vi "dischargetest.vi"(8 "error in":errorcluster, 9 "Serial Configuration":T1={"Baud Rate"=9600, "Parity"=0, "Data Bits"=8, "Stop Bits"=10, "Flow Control"=0} {"Flow Control" items=["None", "XON/XOFF", "RTS/CTS", "XON/XOFF & RTS/CTS", "DTR/DSR", "XON/XOFF & DTR/DSR"]; "Stop Bits" items=["1.0"=10, "1.5"=15, "2.0"=20]; "Data Bits" items=["7"=7, "8"=8]; "Parity" items=["None", "Odd", "Even", "Mark", "Space"]; "Baud Rate" items=["300"=300, "600"=600, "1200"=1200, "2400"=2400, "4800"=4800, "9600"=9600, "19200"=19200]}, 11 "VISA resource name":refnum<visa-resource-name>) -> ()   [LabVIEW 2020]
uses:
  <instrlib>/IT-M3400/IT-M3400.lvlib
panel:
  out "Read Current(A)":dbl format="%.2g"
  out "Read Voltage(V)":dbl format="%.2g"
  in  "stop":bool
  in  "Save File(1-10)":u8=1 min=1 max=10 step=1
  in  "Stop Time(s)":dbl
  in  "Stop Capacity(Ah)":dbl
  in  "Stop Current(A)":dbl
  in  "Stop Voltage(V)":dbl
  in  "Battery Mode":u8(ring) items=["Charge", "Discharge"]
  in  "Discharge Current(A)":dbl
  in  "Discharge Voltage(V)":dbl
  in  "Channel":i32(ring)=1 items=["Channel 1"=1, "Channel 2"=2, "Channel 3"=3, "Channel 4"=4, "Channel 5"=5, "Channel 6"=6, "Channel 7"=7, "Channel 8"=8, "Channel 8"=9, "Channel 10"=10, "Channel 11"=11, "Channel 12"=12, "Channel 13"=13, "Channel 14"=14, "Channel 15"=15, "Channel 16"=16]
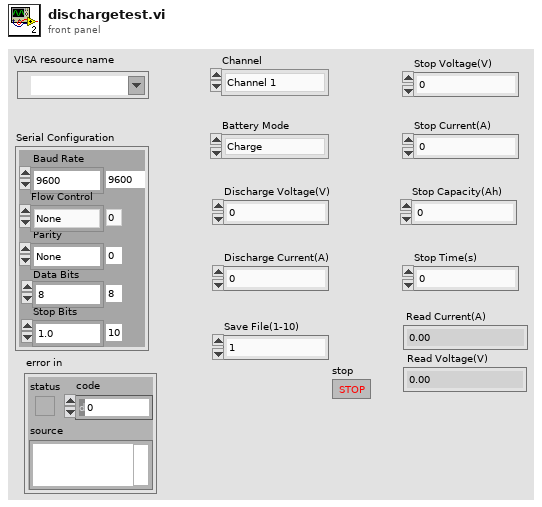
[diagram p1: front panel]
types:
  T1 = cluster{"Baud Rate":u32, "Parity":u16, "Data Bits":u16, "Stop Bits":u16, "Flow Control":u16}
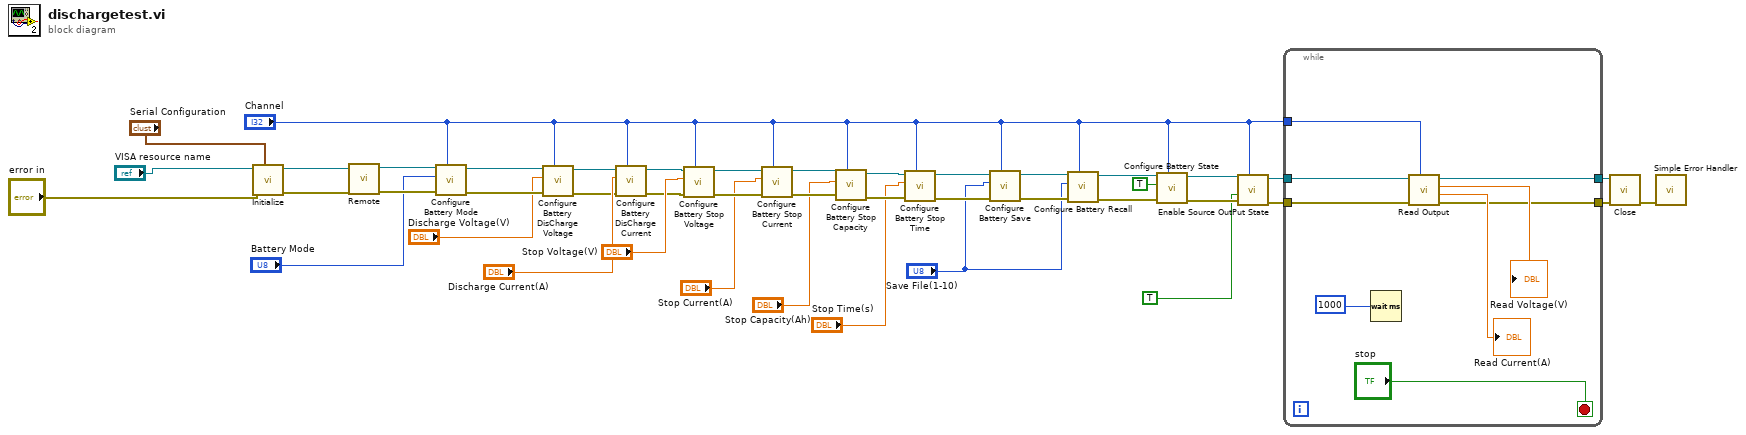
[diagram p0: block diagram]
diagram:
  n1 = call <instrlib>:"Initialize.vi"("Serial Configuration"="Serial Configuration", "error in"="error in", "VISA resource name"="VISA resource name") -> ("error out"=w27:errorcluster, "VISA resource name out"=w28:refnum<visa-resource-name>)  [unwired: 7 in]
  n2 = call <instrlib>:"Remote.vi"("error in"=w27, "VISA resource name"=w28) -> ("error out"=w42:errorcluster, "VISA resource name out"=w43:refnum<visa-resource-name>)  [unwired: 8 in]
  n3 = call <instrlib>:"Configure Battery Mode.vi"("Channel"="Channel", "error in"=w42, "Battery Mode"="Battery Mode", "VISA resource name"=w43) -> ("error out"=w9:errorcluster, "VISA resource name out"=w10:refnum<visa-resource-name>)  [unwired: 6 in]
  n4 = call <instrlib>:"Configure Battery DisCharge Voltage.vi"("Channel"="Channel", "error in"=w9, "Discharge Voltage(V)"="Discharge Voltage(V)", "VISA resource name"=w10) -> ("error out"=w5:errorcluster, "VISA resource name out"=w6:refnum<visa-resource-name>)  [unwired: 6 in]
  n5 = call <instrlib>:"Configure Battery DisCharge Current.vi"("Channel"="Channel", "error in"=w5, "Discharge Current(A)"="Discharge Current(A)", "VISA resource name"=w6) -> ("error out"=w3:errorcluster, "VISA resource name out"=w4:refnum<visa-resource-name>)  [unwired: 6 in]
  n6 = call <instrlib>:"Configure Battery Stop Voltage.vi"("Channel"="Channel", "error in"=w3, "Stop Voltage(V)"="Stop Voltage(V)", "VISA resource name"=w4) -> ("error out"=w40:errorcluster, "VISA resource name out"=w41:refnum<visa-resource-name>)  [unwired: 6 in]
  n7 = call <instrlib>:"Configure Battery Stop Current.vi"("Channel"="Channel", "error in"=w40, "Stop Current(A)"="Stop Current(A)", "VISA resource name"=w41) -> ("error out"=w38:errorcluster, "VISA resource name out"=w39:refnum<visa-resource-name>)  [unwired: 6 in]
  n8 = call <instrlib>:"Configure Battery Stop Capacity.vi"("Channel"="Channel", "error in"=w38, "Stop Capacity(Ah)"="Stop Capacity(Ah)", "VISA resource name"=w39) -> ("error out"=w36:errorcluster, "VISA resource name out"=w37:refnum<visa-resource-name>)  [unwired: 6 in]
  n9 = call <instrlib>:"Configure Battery Stop Time.vi"("Channel"="Channel", "error in"=w36, "Stop Time(S)"="Stop Time(s)", "VISA resource name"=w37) -> ("error out"=w34:errorcluster, "VISA resource name out"=w35:refnum<visa-resource-name>)  [unwired: 6 in]
  n10 = call <instrlib>:"Configure Battery Save.vi"("Channel"="Channel", "error in"=w34, "File"="Save File(1-10)", "VISA resource name"=w35) -> ("error out"=w24:errorcluster, "VISA resource name out"=w25:refnum<visa-resource-name>)  [unwired: 6 in]
  n11 = call <instrlib>:"Configure Battery Recall.vi"("Channel"="Channel", "error in"=w24, "File"="Save File(1-10)", "VISA resource name"=w25) -> ("error out"=w22:errorcluster, "VISA resource name out"=w23:refnum<visa-resource-name>)  [unwired: 6 in]
  n12 = call <instrlib>:"Configure Battery State.vi"("Channel"="Channel", "error in"=w22, "State"=TRUE, "VISA resource name"=w23) -> ("error out"=w19:errorcluster, "VISA resource name out"=w20:refnum<visa-resource-name>)  [unwired: 6 in]
  n13 = call <instrlib>:"Enable Source OutPut State.vi"("Channel"="Channel", "error in"=w19, "State"=TRUE ("Enable Output|Intput"), "VISA resource name"=w20) -> ("error out"=w13:errorcluster, "VISA resource name out"=w14:refnum<visa-resource-name>)  [unwired: 6 in]
  n14 = while {
    tunnel: w14 -> [w49]
    tunnel: w13 -> [w48]
    tunnel: "Channel" -> [w45]
    tunnel: [w47] -> w12
    tunnel: [w46] -> w11
    stop <- "stop" stop-if-true
    n15 = Wait (ms)(milliseconds to wait=1000) -> ()  [unwired: 1 out]
    n16 = call <instrlib>:"Read Output.vi"("Channel"=w45, "error in"=w48, "VISA resource name"=w49) -> ("error out"=w46:errorcluster, "Read Current(A)"=→"Read Current(A)":dbl, "Read Voltage(V)"=→"Read Voltage(V)":dbl, "VISA resource name out"=w47:refnum<visa-resource-name>)  [unwired: 5 in]
  }
  n17 = call <instrlib>:"Close.vi"("error in"=w11, "VISA resource name"=w12) -> ("error out"=w16:errorcluster)  [unwired: 9 in]
  n18 = call <vilib>:"Simple Error Handler.vi"("error in (no error)"=w16) -> ()  [unwired: 4 in, 5 out]
